vi "File_Modified_Since_Check.vi"(6 "error in":errorcluster, 7 "mode":string(combo)="Check Modification", 9 "File Path":path) -> (1 "modifiedSinceRead":bool, 2 "modifiedSinceCheck":bool)   [LabVIEW 2021]
panel:
  out "lastRead":timestamp[](array[timestamp])
  out "lastCheck":timestamp[](array[timestamp])
  out "lastMod":timestamp[](array[timestamp])
  out "trackedPaths":path[](array[path])
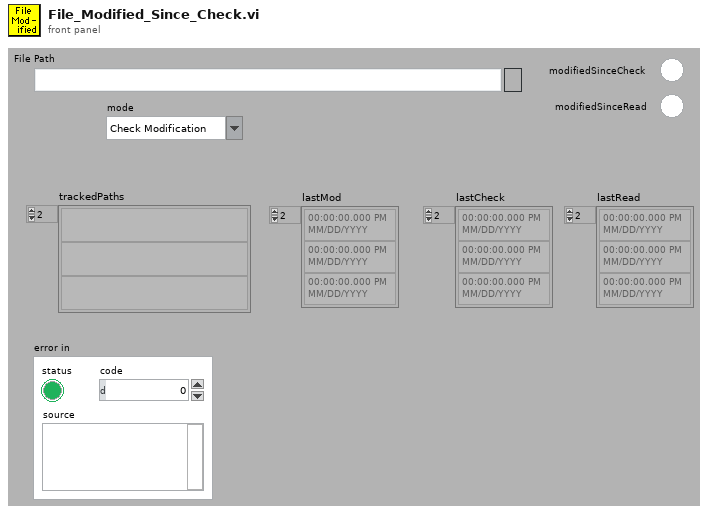
[diagram p1: front panel]
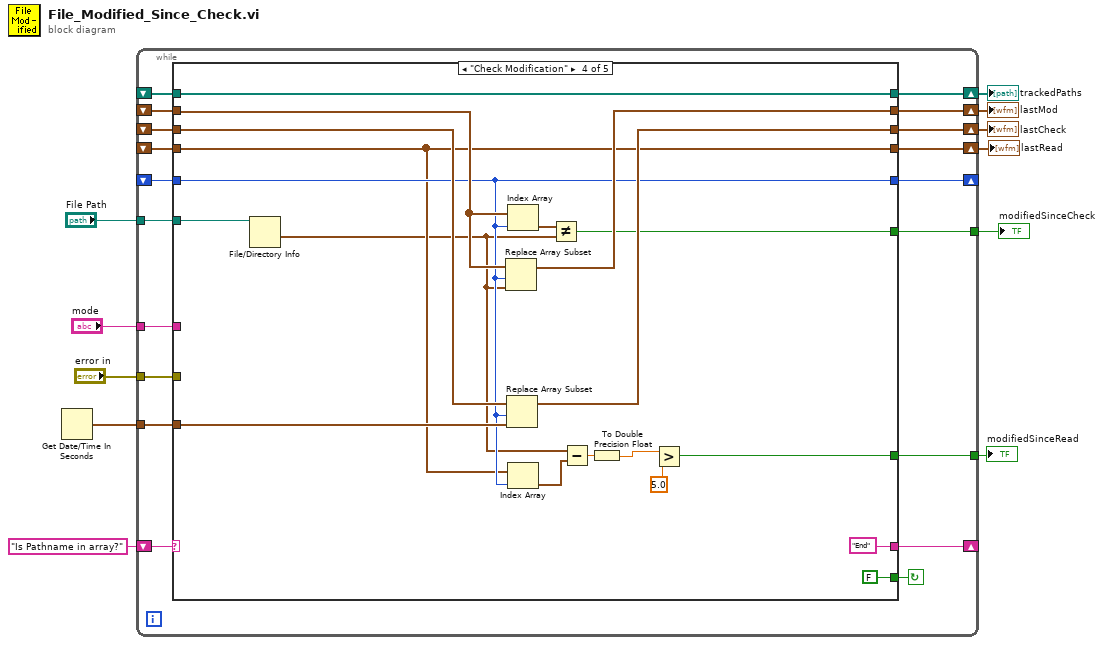
[diagram p0: block diagram]
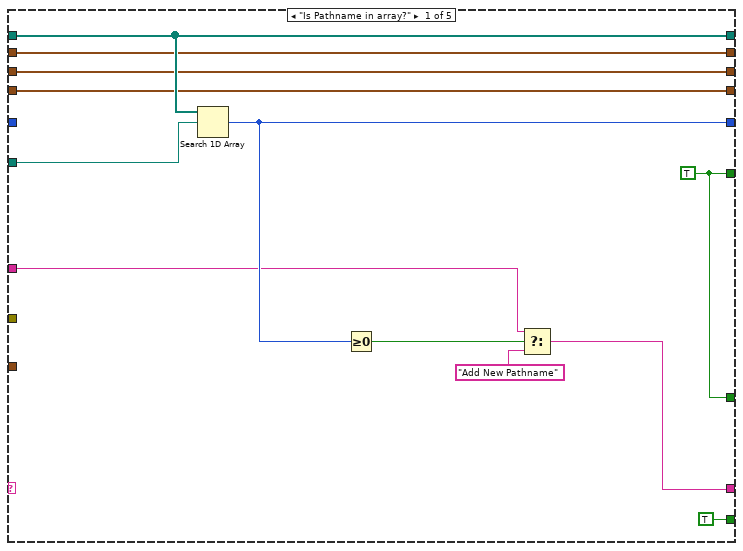
[diagram p2: hidden frame]
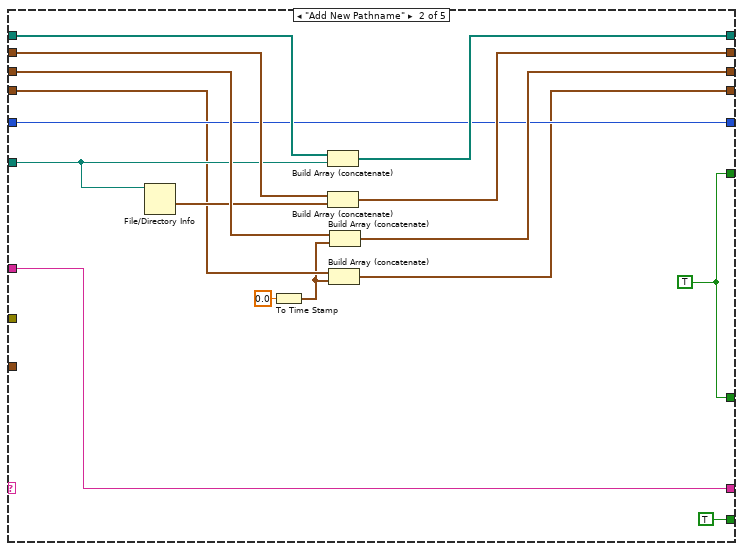
[diagram p3: hidden frame]
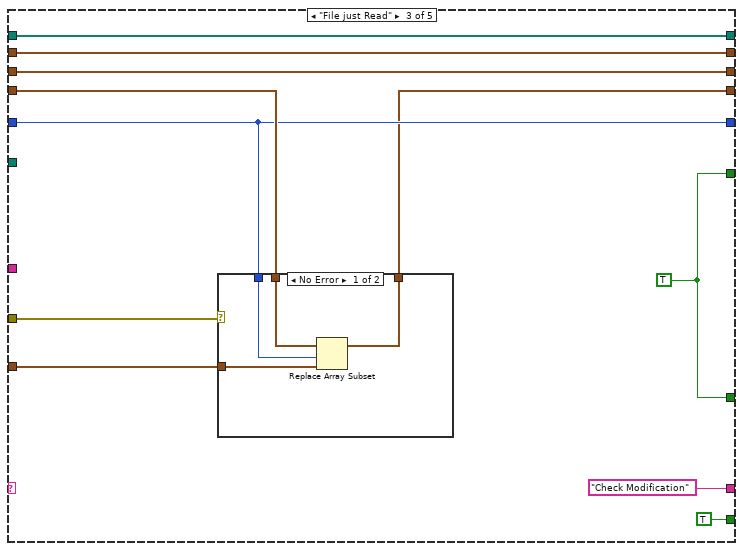
[diagram p4: hidden frame]
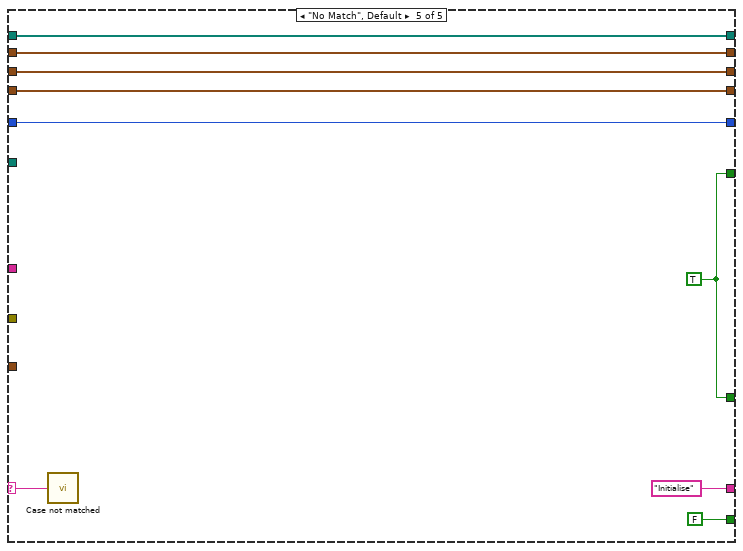
[diagram p6: hidden frame]
diagram:
  n1 = Get Date/Time In Seconds() -> (seconds since 1Jan1904=w9:timestamp)
  n2 = while {
    tunnel: [w17] -> w11
    shift-left: _ -> [w21]
    shift-right: [w20] -> _
    tunnel: w9 -> [w22]
    tunnel: "File Path" -> [w26]
    shift-left: _ -> [w24]
    shift-right: [w18] -> w6
    shift-left: _ -> [w25]
    shift-right: [w19] -> w7
    shift-left: _ -> [w27]
    shift-right: [w23] -> w8
    shift-left: "Is Pathname in array?" ("f") -> [w28]
    shift-right: [w29] -> _
    shift-right: [w15] -> w5
    shift-left: _ -> [w16]
    tunnel: [w14] -> w4
    tunnel: "mode" -> [w13]
    tunnel: "error in" -> [w12]
    stop <- w30 continue-if-true
    n3 = case shown="\"Check Modification\"" w28 {
      selector: w28 -> [_ _ _ _ w96]
      tunnel: [TRUE TRUE TRUE FALSE FALSE] -> w30
      tunnel: [w35 w44 "Check Modification" "End" "Initialise"] -> w29
      tunnel: w27 -> [w40 w57 w67 w91 w100]
      tunnel: w26 -> [w41 w51 _ w87 _]
      tunnel: w25 -> [w39 w56 w66 w85 w99]
      tunnel: w24 -> [w38 w55 w65 w89 w98]
      tunnel: [w40 w54 w67 w91 w100] -> w23
      tunnel: w22 -> [_ _ w62 w90 _]
      tunnel: w21 -> [_ w49 w63 w81 w97]
      tunnel: [w37 w49 w63 w81 w97] -> w20
      tunnel: [w39 w53 w66 w86 w99] -> w19
      tunnel: [w38 w52 w65 w88 w98] -> w18
      tunnel: [w32 w45 w60 w77 w94] -> w17
      tunnel: w16 -> [w33 w48 w64 w80 w95]
      tunnel: [w33 w47 w61 w80 w95] -> w15
      tunnel: [w32 w45 w60 w83 w94] -> w14
      tunnel: w13 -> [w31 w44 _ _ _]
      tunnel: w12 -> [_ _ w59 _ _]
      frame "Is Pathname in array?" {
        w32 = TRUE
        n4 = Search 1D Array(1D array=w40, element=w41) -> (index of element=w37:i32)  [unwired: 1 out]
        n5 = Greater Or Equal To 0?(x=w37) -> (x >= 0?=w36:bool)
        n6 = Select(t=w31, s=w36, f="Add New Pathname") -> (s? t:f=w35:string)
      }
      frame "Add New Pathname" {
        w45 = TRUE
        n7 = File/Directory Info(path=w51) -> (last mod=w50:timestamp)  [unwired: 1 in, 6 out]
        n8 = To Time Stamp(1:0.0) -> (0:w43:timestamp)
        n9 = Build Array (concatenate)(w57, w51) -> (w54:path[])
        n10 = Build Array (concatenate)(w56, w50) -> (w53:timestamp[])
        n11 = Build Array (concatenate)(w48, w43) -> (w47:timestamp[])
        n12 = Build Array (concatenate)(w55, w43) -> (w52:timestamp[])
      }
      frame "File just Read" {
        w60 = TRUE
        n13 = case shown="No Error" w59 {
          tunnel: w64 -> [w73 w74]
          tunnel: w63 -> [w72 _]
          tunnel: w62 -> [w71 _]
          tunnel: [w70 w74] -> w61
          frame No Error {
            n14 = Replace Array Subset(array=w73, new element=w71, index=w72) -> (w70:timestamp[])
          }
          frame Error {
          }
        }
      }
      frame "Check Modification" {
        n15 = File/Directory Info(path=w87) -> (last mod=w79:timestamp)  [unwired: 1 in, 6 out]
        n16 = Replace Array Subset(array=w85, new element=w79, index=w81) -> (w86:timestamp[])
        n17 = Replace Array Subset(array=w89, new element=w90, index=w81) -> (w88:timestamp[])
        n18 = Index Array(array=w85, index=w81) -> (element=w84:timestamp)
        n19 = Index Array(array=w80, index=w81) -> (element=w82:timestamp)
        n20 = Not Equal?(x=w84, y=w79) -> (x != y?=w83:bool)
        n21 = Subtract(x=w79, y=w82) -> (x-y=w78:dbl)
        n22 = To Double Precision Float(number=w78) -> (double precision float=w76:dbl)
        n23 = Greater?(x=w76, y=5.0) -> (0:w77:bool)
      }
      frame "No Match", Default {
        w94 = TRUE
        n24 = call "Case not matched.vi"("Case Name not Matched"=w96) -> ()
      }
    }
  }
  "modifiedSinceRead" <- w11
  "trackedPaths" <- w8
  "lastMod" <- w7
  "lastCheck" <- w6
  "lastRead" <- w5
  "modifiedSinceCheck" <- w4
